vi "EigenValue_Hierarchy.vi"(7 "NumCh to be Selected":i32=3, 10 "Weight Array (Wx)":dbl[][](array[numeric]), 11 "EigenValues":dbl[](array[numeric])) -> (3 "WL":dbl[][](array[numeric]))   [LabVIEW 2014]
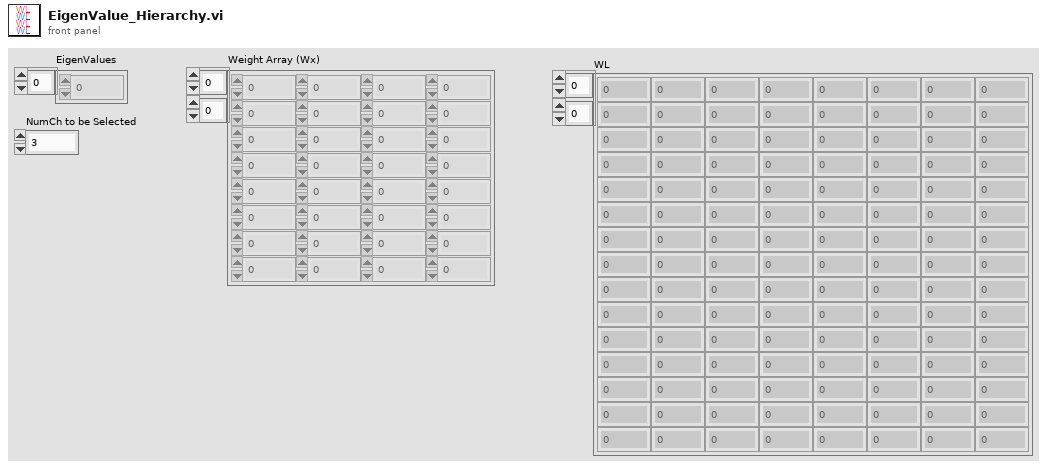
[diagram p1: front panel]
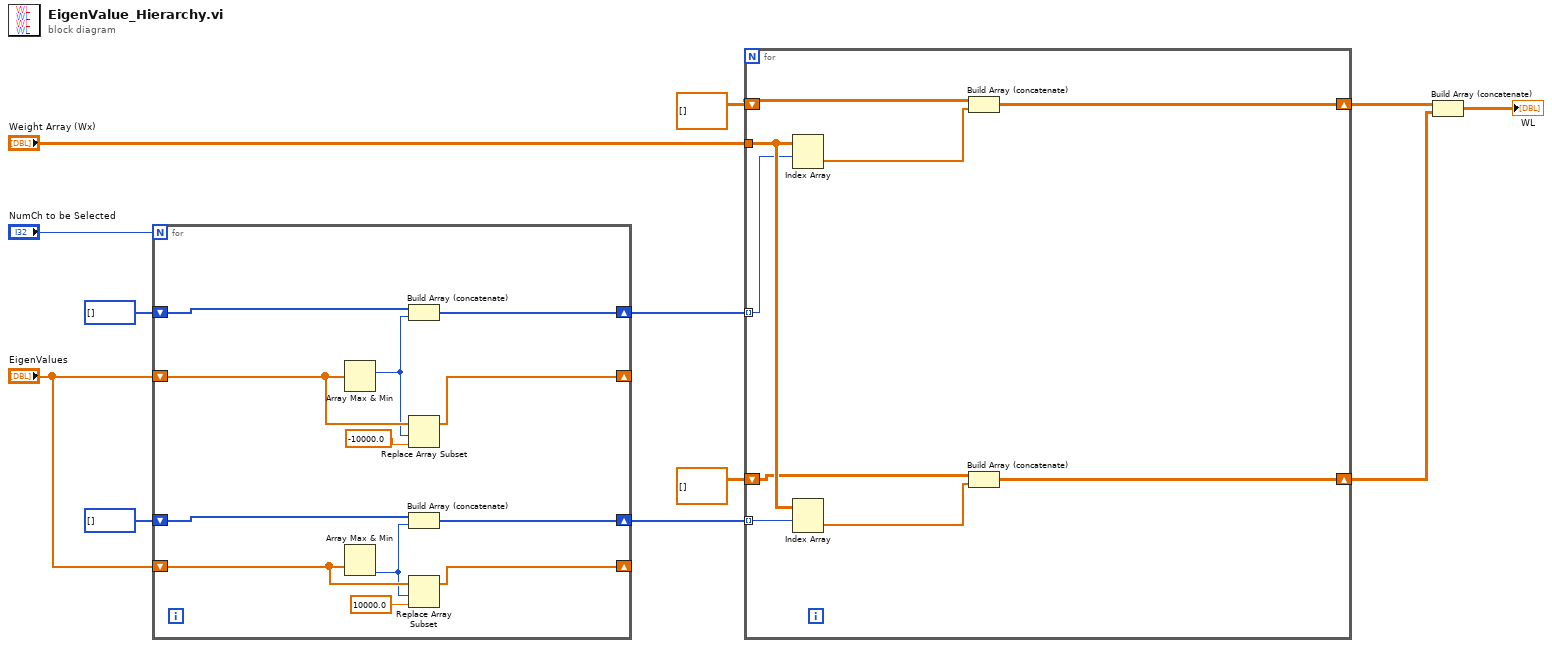
[diagram p0: block diagram]
diagram:
  n1 = for {
    N: "NumCh to be Selected" -> [_]
    shift-right: [w19] -> _
    shift-left: "EigenValues" -> [w22]
    shift-right: [w13] -> _
    shift-left: "EigenValues" -> [w15]
    shift-right: [w24] -> w7
    shift-left: i32[] [] -> [w23]
    shift-right: [w18] -> w6
    shift-left: i32[] [] -> [w17]
    n2 = Array Max & Min(array=w22) -> (max index (indices)=w21:i32)  [unwired: 3 out]
    n3 = Array Max & Min(array=w15) -> (min index (indices)=w14:i32)  [unwired: 3 out]
    n4 = Build Array (concatenate)(w23, w21) -> (w24:i32[])
    n5 = Replace Array Subset(array=w22, new element=-10000.0 ("new element/subarray"), index=w21) -> (w19:dbl[])
    n6 = Build Array (concatenate)(w17, w14) -> (w18:i32[])
    n7 = Replace Array Subset(array=w15, new element=10000.0 ("new element/subarray"), index=w14) -> (w13:dbl[])
  }
  n8 = for {
    tunnel: "Weight Array (Wx)" -> [w33]
    tunnel: w7 -> [w32] mode=indexing
    tunnel: w6 -> [w31] mode=indexing
    shift-right: [w29] -> w3
    shift-left: dbl[][] [] -> [w28]
    shift-right: [w26] -> w2
    shift-left: dbl[][] [] -> [w25]
    n9 = Index Array(array=w33, index (row)=w32) -> (element=w30:dbl[])  [unwired: 1 in]
    n10 = Index Array(array=w33, index (row)=w31) -> (element=w27:dbl[])  [unwired: 1 in]
    n11 = Build Array (concatenate)(w28, w30) -> (w29:dbl[][])
    n12 = Build Array (concatenate)(w25, w27) -> (w26:dbl[][])
  }
  n13 = Build Array (concatenate)(w3, w2) -> (→"WL":dbl[][])
